vi "GenColumnHeaders.vi"(11 "Array in":cluster{string, i32}[](array[cluster])) -> (1 "Starting Column of Each Variable":i32[](array[numeric]), 2 "Total Number of Columns":i32, 3 "String+\\n":string)   [LabVIEW 2016]
uses:
  <vilib>/AuZn/auzn custom VIs/AuZnCustomVI.lvlib
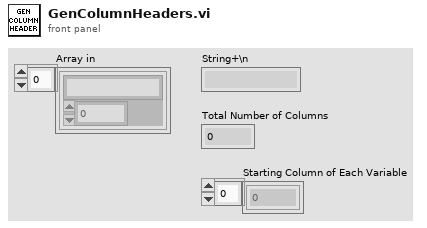
[diagram p1: front panel]
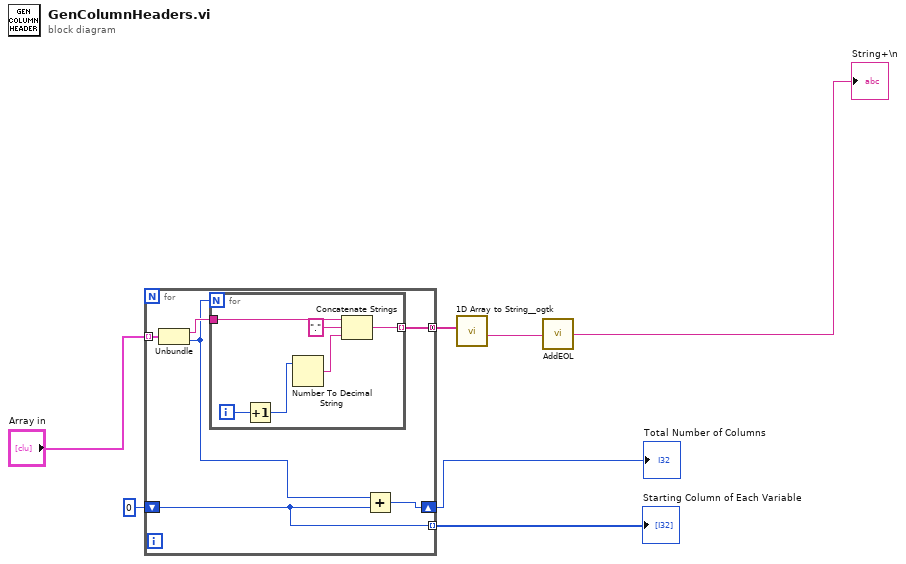
[diagram p0: block diagram]
diagram:
  n1 = for {
    tunnel: [w13] -> w1 mode=concatenating
    tunnel: "Array in" -> [w11] mode=indexing
    shift-right: [w9] -> w7
    shift-left: 0 -> [w8]
    tunnel: [w8] -> w6 mode=indexing
    n2 = Unbundle(w11) -> (w12:string, w10:i32)
    n3 = for {
      N: w10 -> [_]
      tunnel: w12 -> [w19]
      tunnel: [w14] -> w13 mode=indexing
      i -> [w16]
      n4 = Increment(x=w16) -> (x+1=w15:i32)
      n5 = Number To Decimal String(number=w15) -> (decimal integer string=w17:string)  [unwired: 1 in]
      n6 = Concatenate Strings(w19, ".", w17) -> (w14:string)
    }
    n7 = Add(x=w10, y=w8) -> (x+y=w9:i32)
  }
  "Total Number of Columns" <- w7
  "Starting Column of Each Variable" <- w6
  n8 = call <userlib>:"1D Array to String__ogtk.vi"("Array of Strings"=w1) -> ("delimited string"=w2:string)  [unwired: 10 in]
  n9 = call <vilib>:"AddEOL.vi"("String in"=w2) -> ("String+\\n"=→"String+\\n":string)
